vi "Load CSV 1D data.vi"(8 "error in":errorcluster, 11 "start path":path=path "") -> (0 "error out":errorcluster, 2 "data":dbl[](array[numeric]), 3 "last path":path caption="start path")   [LabVIEW 2013]
doc: "Loads CSV 1D vector of numbers. Auto guessing decimal and value separators. Has open dialog integrated."
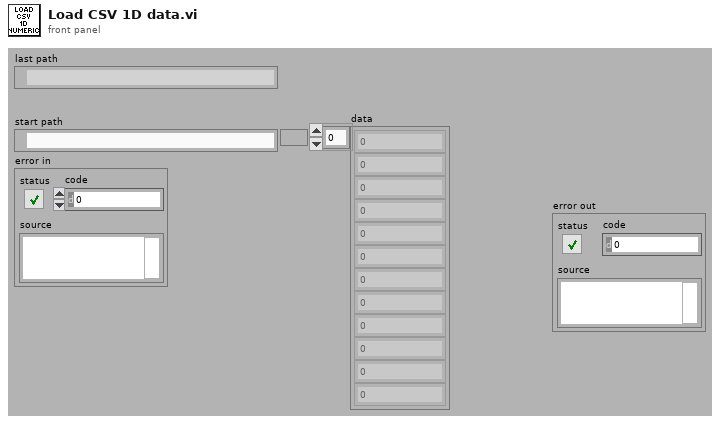
[diagram p1: front panel]
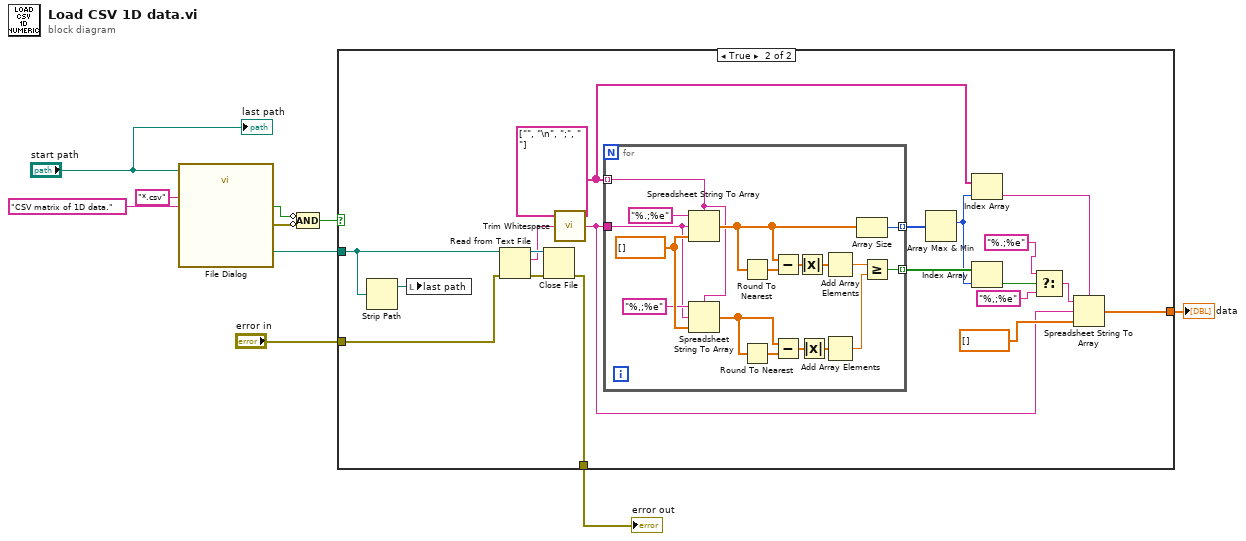
[diagram p0: block diagram]
diagram:
  n1 = call "File Dialog"("start path"="start path", "pattern (all files)"="*.csv", "pattern label"="CSV matrix of 1D data.") -> ("selected path"=w4:path, "cancelled"=w6:bool, "error out"=w7:errorcluster)  [unwired: 9 in, 1 out]
  n2 = Compound Arithmetic op=AND(invert w6, invert w7) -> (w5:bool)
  n3 = case shown="True" w5 {
    tunnel: w4 -> [_ w29]
    tunnel: [_ w15] -> w3
    tunnel: "error in" -> [w11 w14]
    tunnel: [w11 w13] -> w1
    frame False {
    }
    frame True {
      w23 = string[] ["", "\n", ";", " "]
      n4 = Strip Path(path=w29) -> (stripped path=w30:path)  [unwired: 1 out]
      n5 = local write "last path"(w30) -> ()
      n6 = Read from Text File(file (use dialog)=w29, error in=w14) -> (refnum out=w28:refnum<file>, text=w21:string, error out=w27:errorcluster)  [unwired: 2 in, 1 out]
      n7 = Close File(refnum=w28, error in=w27) -> (error out=w13:errorcluster)  [unwired: 1 out]
      n8 = call <vilib>:"Trim Whitespace.vi"("string"=w21) -> ("trimmed string"=w12:string)  [unwired: 1 in]
      n9 = for {
        tunnel: w23 -> [w41] mode=indexing
        tunnel: w12 -> [w39]
        tunnel: [w46] -> w26 mode=indexing
        tunnel: [w31] -> w25 mode=indexing
        w42 = dbl[] []
        n10 = Spreadsheet String To Array(delimiter (Tab)=w41, format string="%.;%e", spreadsheet string=w39, array type (2D Dbl)=w42) -> (array=w44:dbl[])
        n11 = Spreadsheet String To Array(delimiter (Tab)=w41, format string="%,;%e", spreadsheet string=w39, array type (2D Dbl)=w42) -> (array=w36:dbl[])
        n12 = Round To Nearest(number=w44) -> (nearest integer value=w45:dbl[])
        n13 = Round To Nearest(number=w36) -> (nearest integer value=w37:dbl[])
        n14 = Subtract(x=w44, y=w45) -> (x-y=w43:dbl[])
        n15 = Subtract(x=w36, y=w37) -> (x-y=w38:dbl[])
        n16 = Absolute Value(x=w43) -> (abs(x)=w35:dbl[])
        n17 = Absolute Value(x=w38) -> (abs(x)=w34:dbl[])
        n18 = Add Array Elements(numeric array=w35) -> (sum=w33:dbl)
        n19 = Add Array Elements(numeric array=w34) -> (sum=w32:dbl)
        n20 = Array Size(array=w44) -> (size(s)=w46:i32)
        n21 = Greater Or Equal?(x=w33, y=w32) -> (x >= y?=w31:bool)
      }
      n22 = Array Max & Min(array=w26) -> (max index (indices)=w24:i32)  [unwired: 3 out]
      n23 = Index Array(array=w23, index=w24) -> (element=w22:string)
      n24 = Index Array(array=w25, index=w24) -> (element=w19:bool)
      n25 = Select(t="%.;%e" ("format string"), s=w19, f="%,;%e" ("format string")) -> (s? t:f=w16:string)
      n26 = Spreadsheet String To Array(delimiter (Tab)=w22, format string=w16, spreadsheet string=w12, array type (2D Dbl)=dbl[] []) -> (array=w15:dbl[])
    }
  }
  "data" <- w3
  "error out" <- w1
  "last path" <- "start path"
